vi "XIPIN_SMPTE_2022-1_2_Video_over_IP_Receiver_2_0.vi"   [LabVIEW 2017]
doc: "The Xilinx LogiCORE IP SMPTE 2022-1/2 Video over IP Receiver is a module for broadcast applications that requires bridging between SMPTE video connectivity standards (ASI) and 1Gb/s networks. The module is capable of recovering IP packets lost to network transmission errors and ensure the picture quality of uncompressed, high bandwidth professional video.\n------------------------------------\n<b>Need License</b> : Yes\n<b>Interface</b> : AXI4 AXI4-Stream"
uses:
  <vilib>/rvi/XilinxIP/XIPIN_XNode/niFpgaXIPIN.xnode
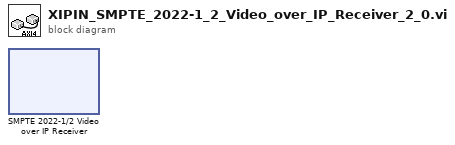
[diagram p0: block diagram]
diagram:
  n1 = xnode ("SMPTE 2022-1/2 Video over IP Receiver")() -> ()
